vi "read_params.vi"(8 "error in (no error)":errorcluster, 11 "LinearDiscriminantAnalysis in":refnum<class "LinearDiscriminantAnalysis.lvclass">) -> (0 "error out":errorcluster, 2 "params":T1={"solver"="svd", "shrinkage"={"shrinkage_type"="None", "shrinkage_float"=0.0}, "priors"={"priors_type"="None", "priors_list"=[]}, "n_components"={"n_components_type"="None", "n_components_int"=0.0}, "store_covariance"=FALSE, "tol"=0.0001}, 3 "LinearDiscriminantAnalysis out":refnum<class "LinearDiscriminantAnalysis.lvclass">)   [LabVIEW 2020, in "LinearDiscriminantAnalysis.lvclass"]
uses:
  LinearDiscriminantAnalysis.lvclass
  Controls/linear_discriminant_analysis_params.ctl
  LinearDiscriminantAnalysis.lvclass/LinearDiscriminantAnalysis.ctl
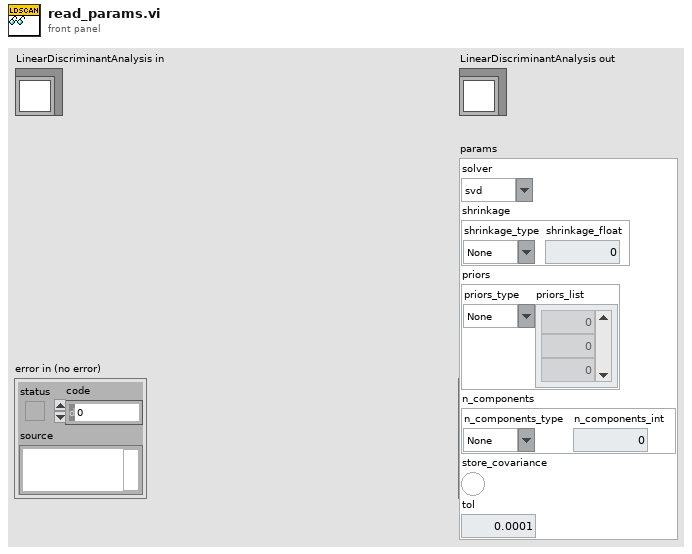
[diagram p1: front panel]
types:
  T1 = typedef "linear_discriminant_analysis_params.ctl" = cluster{"solver":string, "shrinkage":cluster{"shrinkage_type":string, "shrinkage_float":dbl}, "priors":cluster{"priors_type":string, "priors_list":dbl[]}, "n_components":cluster{"n_components_type":string, "n_components_int":dbl}, "store_covariance":bool, "tol":dbl}
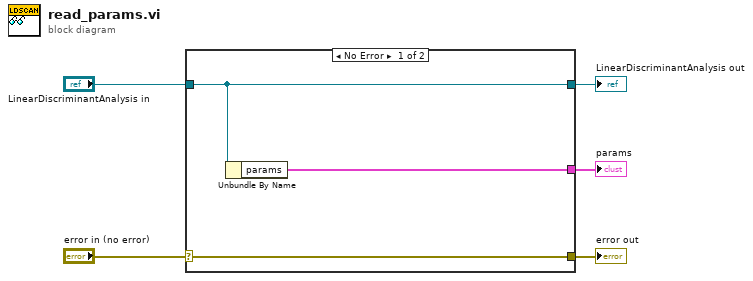
[diagram p0: block diagram]
diagram:
  n1 = case shown="No Error" "error in (no error)" {
    selector: "error in (no error)" -> [w8 w9]
    tunnel: [w8 w9] -> w4
    tunnel: [w7 w10] -> w2
    tunnel: "LinearDiscriminantAnalysis in" -> [w7 w10]
    tunnel: [w6 _] -> w1
    frame No Error {
      n2 = Unbundle By Name(w7) -> ("params"=w6:T1)
    }
    frame Error {
    }
  }
  "error out" <- w4
  "LinearDiscriminantAnalysis out" <- w2
  "params" <- w1
